vi "Handle Incoming Packets.vi"(8 "error in (no error)":errorcluster, 9 "SessionMailbox":refnum<queue>, 10 "Incoming Packet":refnum<class "ControlPacket.lvclass">, 11 "Server in":refnum<class "Server.lvclass">) -> (0 "error out":errorcluster, 1 "SessionMailbox out":refnum<queue>, 2 "Outgoing":T1, 3 "Server out":refnum<class "Server.lvclass">)   [LabVIEW 2013, in "MQTT Server.lvlib" / "Server.lvclass"]
uses:
  Server.lvclass
  <vilib>/LabVIEW Open Source Project/MQTT Control Packets/Control Packets/ControlPacket/ControlPacket.lvclass
  <vilib>/LabVIEW Open Source Project/MQTT Connection/MQTT_Base/Base Class/Response -- cluster.ctl
  <vilib>/LabVIEW Open Source Project/MQTT Connection/MQTT_Base/Base Class/MQTT_Base.lvclass
  <vilib>/LabVIEW Open Source Project/MQTT Control Packets/Control Packets/CONNECT/CONNECT.lvclass
  <vilib>/LabVIEW Open Source Project/MQTT Control Packets/Control Packets/CONNACK/Connect Return Code -- enum.ctl
  <vilib>/LabVIEW Open Source Project/MQTT Control Packets/Control Packets/DISCONNECT/DISCONNECT.lvclass
  <vilib>/LabVIEW Open Source Project/MQTT Control Packets/Control Packets/PUBLISH/PUBLISH.lvclass
  <vilib>/LabVIEW Open Source Project/MQTT Control Packets/Control Packets/PUBREL/PUBREL.lvclass
  <vilib>/LabVIEW Open Source Project/MQTT Control Packets/Control Packets/SUBSCRIBE/SUBSCRIBE.lvclass
  <vilib>/LabVIEW Open Source Project/MQTT Control Packets/Control Packets/ControlPacket/ControlPacket.lvclass/ControlPacket.ctl
  <vilib>/LabVIEW Open Source Project/MQTT Control Packets/Control Packets/SUBACK/Subscription Success Code.ctl
  <vilib>/LabVIEW Open Source Project/MQTT Control Packets/Control Packets/ControlPacket/QualityOfService -- enum.ctl
  <vilib>/LabVIEW Open Source Project/MQTT Control Packets/Control Packets/UNSUBSCRIBE/UNSUBSCRIBE.lvclass
  <vilib>/LabVIEW Open Source Project/MQTT Control Packets/Control Packets/PINGREQ/PINGREQ.lvclass
  <vilib>/LabVIEW Open Source Project/MQTT Control Packets/Control Packets/CONNACK/CONNACK.lvclass
  <vilib>/LabVIEW Open Source Project/MQTT Control Packets/Control Packets/SUBACK/SUBACK.lvclass
  <vilib>/LabVIEW Open Source Project/MQTT Control Packets/Control Packets/PINGRESP/PINGRESP.lvclass
  <vilib>/LabVIEW Open Source Project/MQTT Control Packets/Control Packets/UNSUBACK/UNSUBACK.lvclass
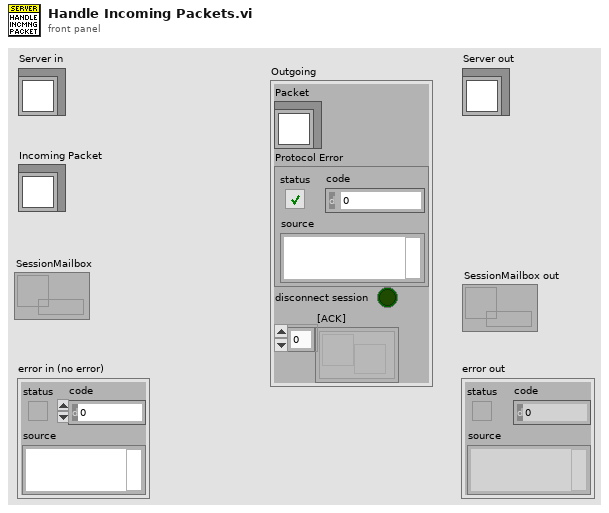
[diagram p1: front panel]
types:
  T1 = typedef "MQTT Base.lvlib/MQTT_Base.lvclass/Response -- cluster.ctl" = cluster{"Packet":refnum<class "ControlPacket.lvclass">, "Protocol Error":errorcluster, "disconnect session":bool, "[ACK]":refnum<notifier>[]}
  T2 = typedef "MQTT_Control_Packets.lvlib/CONNACK.lvclass/Connect Return Code -- enum.ctl" = enum16{"Connection accepted", "Unacceptable protocol version", "Identifier Rejected", "Server Unavailable", "Bad Username or Password", "Not Authorized"}
  T3 = typedef "MQTT_Control_Packets.lvlib/SUBACK.lvclass/Subscription Success Code.ctl" = cluster{"Subscription Failure":bool, "QoS":T4}
  T4 = typedef "MQTT_Control_Packets.lvlib/ControlPacket.lvclass/QualityOfService -- enum.ctl" = enum16{"0 (At Most Once)", "1 (At Least Once)", "2 (Exactly Once)"}
  T5 = typedef "MQTT_Control_Packets.lvlib/ControlPacket.lvclass/Control Packet Type -- enum.ctl" = enum16{"Reserved", "CONNECT", "CONNACK", "PUBLISH", "PUBACK", "PUBREC", "PUBREL", "PUBCOMP", "SUBSCRIBE", "SUBACK", "UNSUBSCRIBE", "UNSUBACK", "PINGREQ", "PINGRESP", "DISCONNECT", "AUTH"}
  T6 = typedef "MQTT_Control_Packets.lvlib/CONNECT.lvclass/ConnectFlags -- cluster.ctl" = cluster{"Reserved":bool, "Clean Session":bool, "Will Flag":bool, "Will QoS 1":bool, "Will QoS 2":bool, "Will Retain":bool, "Password Flag":bool, "User Name Flag":bool}
  T7 = typedef "MQTT_Control_Packets.lvlib/CONNECT.lvclass/ConnectPayload -- cluster.ctl" = cluster{"Will Topic":string, "Will Message":string, "Username":string, "Password":string}
  T8 = typedef "MQTT_Control_Packets.lvlib/SUBSCRIBE.lvclass/Topic Subscription -- cluster.ctl" = cluster{"Topic Filter":string, "QoS":T4}
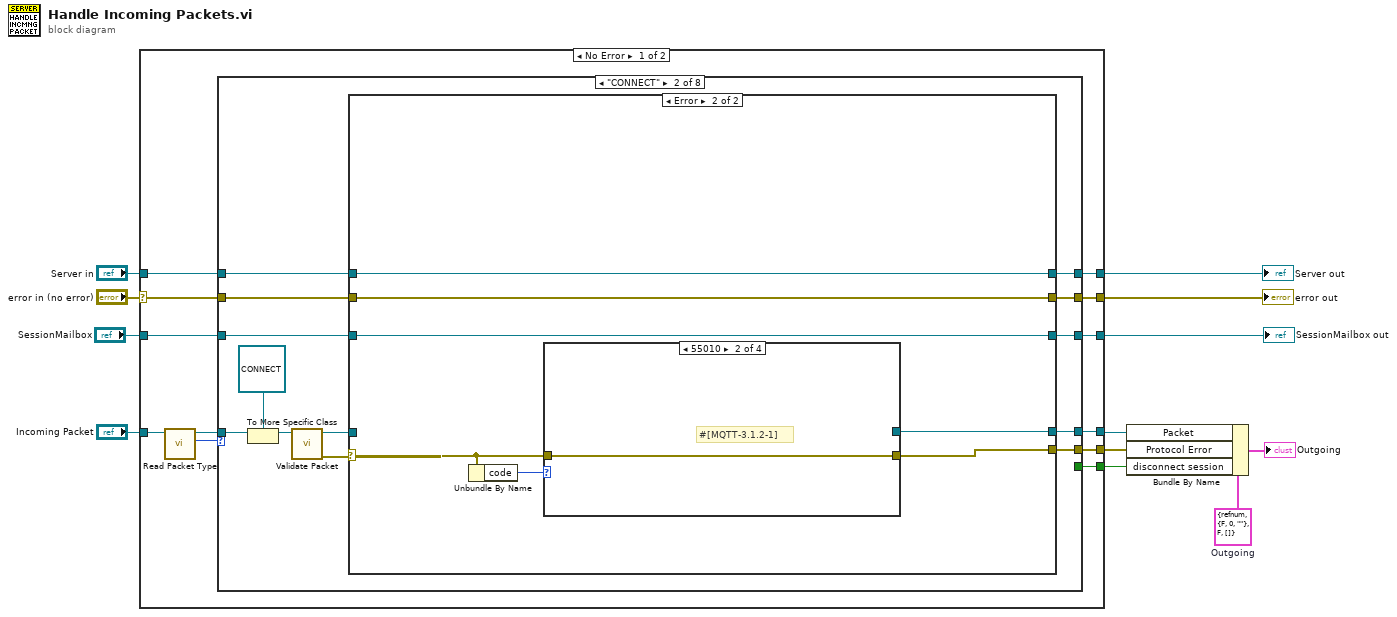
[diagram p0: block diagram]
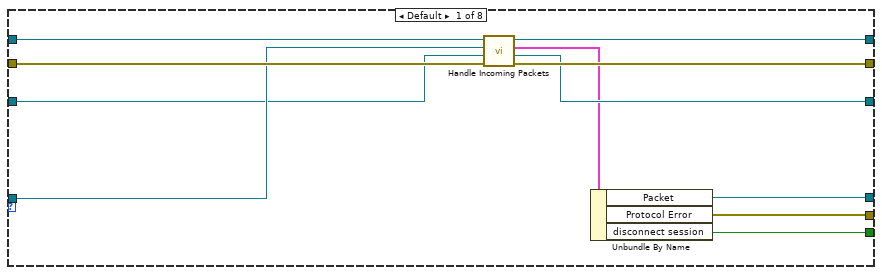
[diagram p2: hidden frame]
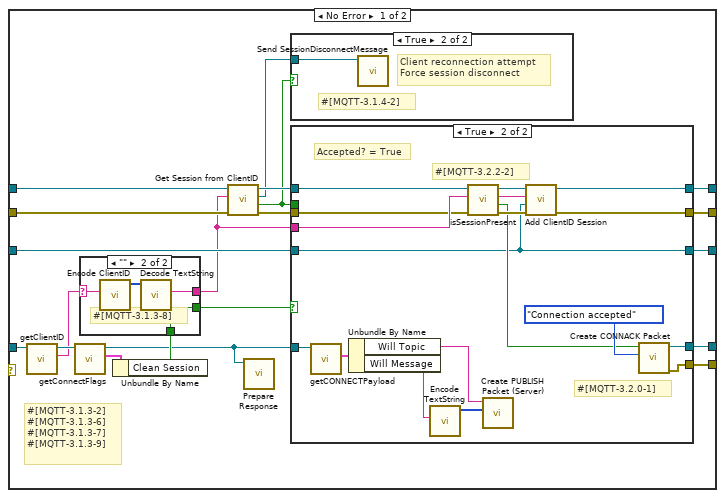
[diagram p3: hidden frame]
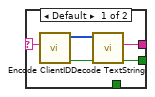
[diagram p4: hidden frame]
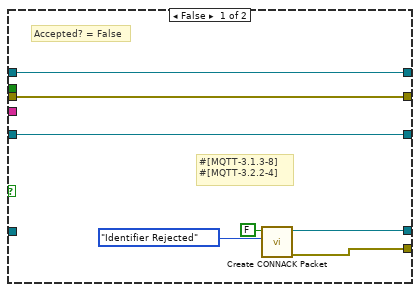
[diagram p6: hidden frame]
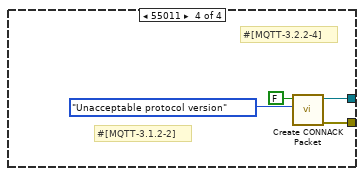
[diagram p9: hidden frame]
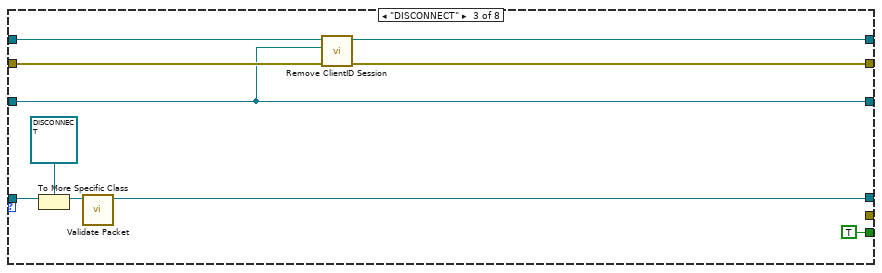
[diagram p10: hidden frame]
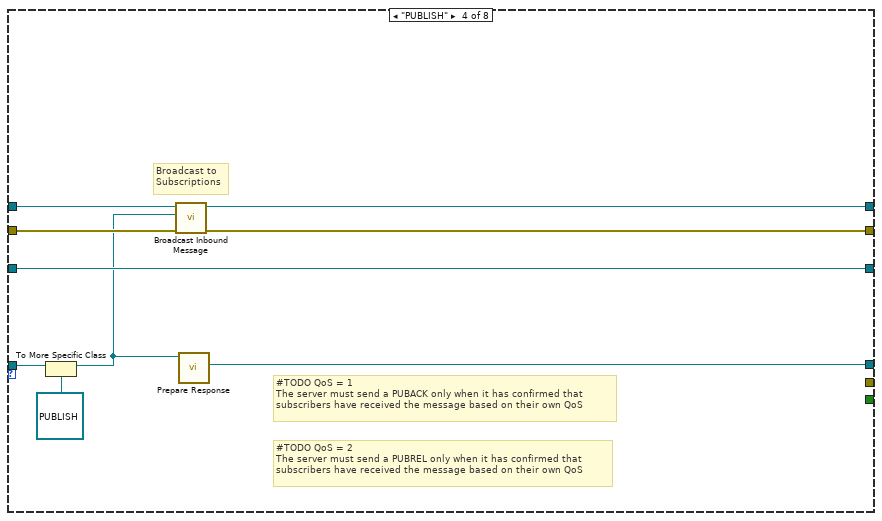
[diagram p11: hidden frame]
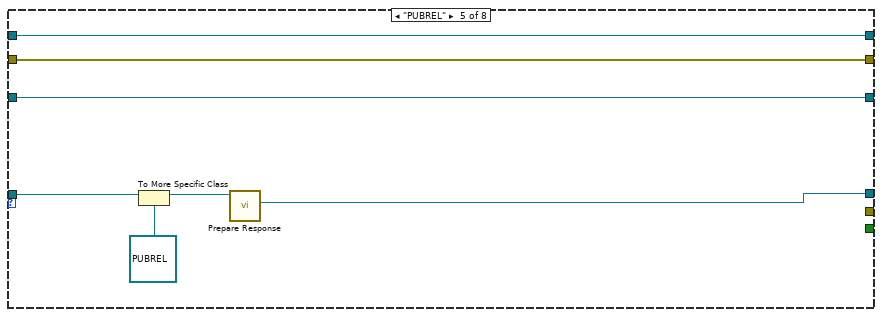
[diagram p12: hidden frame]
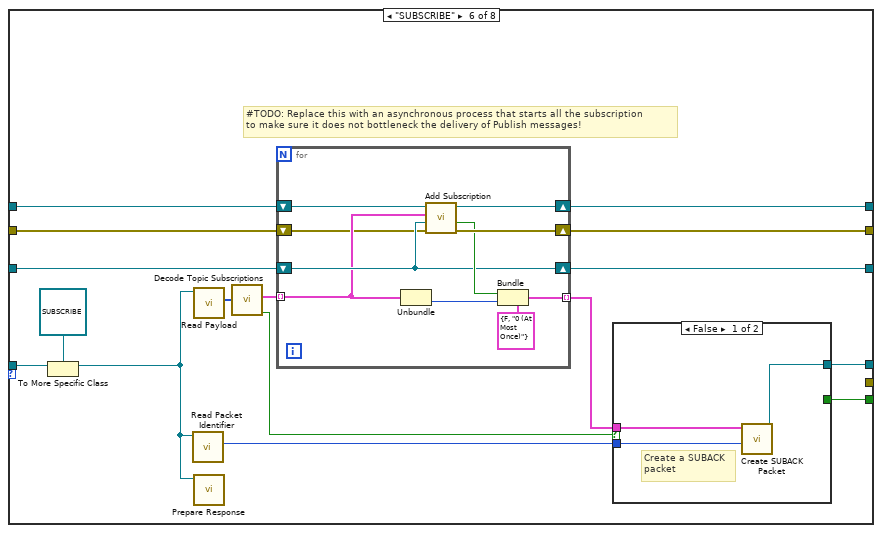
[diagram p13: hidden frame]
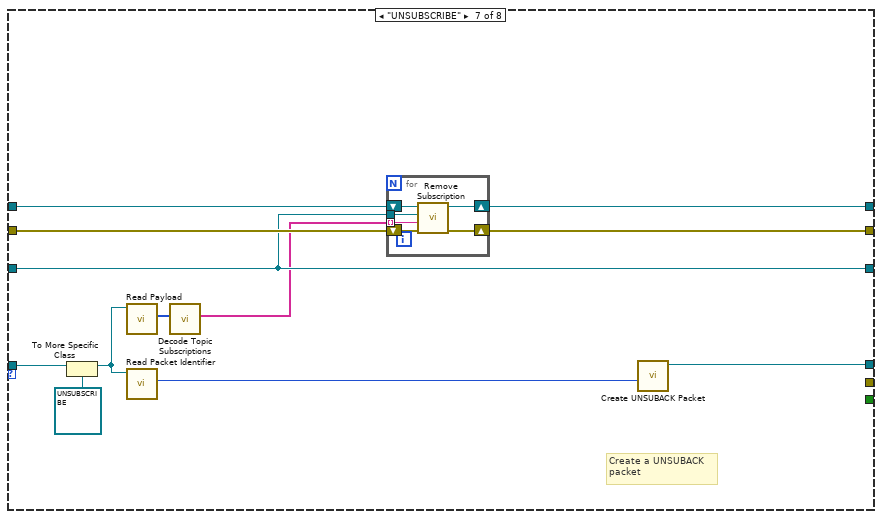
[diagram p15: hidden frame]
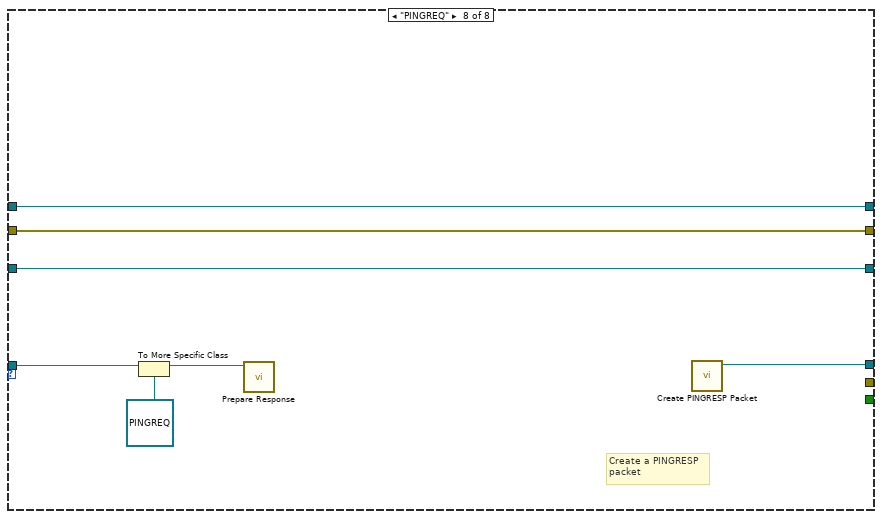
[diagram p16: hidden frame]
diagram:
  w7 = T1 {"Packet"=refnum, "Protocol Error"={"status"=FALSE, "code"=0, "source"=""}, "disconnect session"=FALSE, "[ACK]"=[]}  # Outgoing
  n1 = case shown="No Error" "error in (no error)" {
    selector: "error in (no error)" -> [w22 w200]
    tunnel: [w19 w200] -> w11
    tunnel: [w20 w199] -> w9
    tunnel: "Server in" -> [w21 w199]
    tunnel: "Incoming Packet" -> [w15 _]
    tunnel: [w18 _] -> w6
    tunnel: [w17 _] -> w2
    tunnel: "SessionMailbox" -> [w16 w198]
    tunnel: [w14 w198] -> w1
    tunnel: [w13 _] -> w4
    frame No Error {
      n2 = call <vilib>:"Read Packet Type.vi"("ControlPacket in"=w15) -> ("Control Packet Type"=w24:T5, "ControlPacket out"=w23:refnum<class "ControlPacket.lvclass">)  [unwired: 9 in]
      n3 = case shown="\"CONNECT\"" w24 {
        tunnel: w23 -> [w31 w45 w126 w134 w139 w158 w184 w194]
        tunnel: w22 -> [w33 w42 w121 w132 w141 w148 w180 w196]
        tunnel: w21 -> [w35 w43 w123 w130 w142 w151 w178 w197]
        tunnel: [w34 w40 w122 w129 w142 w150 w177 w197] -> w20
        tunnel: [w32 w41 w120 w131 w141 w149 w179 w196] -> w19
        tunnel: w16 -> [w30 w39 w119 w135 w140 w147 w176 w195]
        tunnel: [w27 w38 w117 w127 w136 w152 w174 w193] -> w18
        tunnel: [w26 w37 _ _ _ _ _ _] -> w17
        tunnel: [w29 w36 w119 w135 w140 w146 w176 w195] -> w14
        tunnel: [w25 _ TRUE ("disconnect session") _ _ w144 _ _] -> w13
        frame Default {
          n4 = call-parent "Handle Incoming Packets.vi"("error in (no error)"=w33, "SessionMailbox"=w30, "Incoming Packet"=w31, "MQTT_Base in"=w35) -> ("error out"=w32:errorcluster, "SessionMailbox out"=w29:refnum<queue>, "Outgoing"=w28:T1, "MQTT_Base out"=w34:refnum<class "Server.lvclass">)  [unwired: 4 in]
          n5 = Unbundle By Name(w28) -> ("Packet"=w27:refnum<class "ControlPacket.lvclass">, "Protocol Error"=w26:errorcluster, "disconnect session"=w25:bool)
        }
        frame "CONNECT" {
          n6 = To More Specific Class(target class=refnum<class "CONNECT.lvclass"> refnum ("CONNECT.lvclass"), reference=w45) -> (specific class reference=w44:refnum<class "CONNECT.lvclass">)  [unwired: 1 in, 1 out]
          n7 = call <vilib>:"Validate Packet.vi"("ControlPacket in"=w44) -> ("error out"=w48:errorcluster, "ControlPacket out"=w47:refnum<class "CONNECT.lvclass">)  [unwired: 9 in]
          n8 = case shown="Error" w48 {
            selector: w48 -> [_ w108]
            tunnel: w47 -> [w68 _]
            tunnel: w43 -> [w64 w107]
            tunnel: w42 -> [w62 w106]
            tunnel: [w66 w106] -> w41
            tunnel: [w67 w107] -> w40
            tunnel: w39 -> [w65 w103]
            tunnel: [w59 w105] -> w38
            tunnel: [w58 w104] -> w37
            tunnel: [w56 w103] -> w36
            frame No Error {
              # "#[MQTT-3.1.3-2]\n#[MQTT-3.1.3-6]\n#[MQTT-3.1.3-7]\n#[MQTT-3.1.3-9]"
              n9 = call <vilib>:"getClientID.vi"("CONNECT in"=w68) -> ("Client ID"=w51:string, "CONNECT out"=w55:refnum<class "CONNECT.lvclass">)  [unwired: 9 in]
              n10 = call <vilib>:"getConnectFlags.vi"("CONNECT in"=w55) -> ("Connect Flags"=w54:T6, "CONNECT out"=w49:refnum<class "CONNECT.lvclass">)  [unwired: 9 in]
              n11 = Unbundle By Name(w54) -> ("Clean Session"=w52:bool)
              n12 = case shown="\"\"" w51 {
                selector: w51 -> [w72 w75]
                tunnel: [w71 w76] -> w53
                tunnel: w52 -> [_ w76]
                tunnel: [w69 w73] -> w50
                frame Default {
                  n13 = call <vilib>:"Encode ClientID.vi"("Client ID (empty: generate new)"=w72) -> ("valid Client ID"=w71:bool, "Length-Prefixed Field"=w70:u8[])  [unwired: 9 in]
                  n14 = call <vilib>:"Decode TextString.vi"("Length-Prefixed Field"=w70) -> ("Text String"=w69:string)  [unwired: 8 in, 2 out]
                }
                frame "" {
                  # "#[MQTT-3.1.3-8]"
                  n15 = call <vilib>:"Encode ClientID.vi"("Client ID (empty: generate new)"=w75) -> ("Length-Prefixed Field"=w74:u8[])  [unwired: 9 in, 1 out]
                  n16 = call <vilib>:"Decode TextString.vi"("Length-Prefixed Field"=w74) -> ("Text String"=w73:string)  [unwired: 8 in, 2 out]
                }
              }
              n17 = call "Get Session from ClientID.vi"("error in (no error)"=w62, "Client ID"=w50, "MQTT Server"=w64) -> ("error out"=w61:errorcluster, "found?"=w57:bool, "SessionMailbox"=w60:refnum<queue>, "MQTT Server"=w63:refnum<class "Server.lvclass">)  [unwired: 5 in]
              n18 = call-dynamic "Prepare Response.vi"("ControlPacket in"=w49) -> ()  [unwired: 7 in, 4 out]
              n19 = case shown="True" w57 {
                tunnel: w60 -> [_ w77]
                frame False {
                }
                frame True {
                  # "#[MQTT-3.1.4-2]"
                  # "Client reconnection attempt\nForce session disconnect"
                  n20 = call "Send SessionDisconnectMessage.vi"("SessionMailbox"=w77) -> ()  [unwired: 10 in, 1 out]
                }
              }
              n21 = case shown="True" w53 {
                tunnel: [w82 w101] -> w67
                tunnel: [w81 w100] -> w66
                tunnel: w65 -> [w78 w90]
                tunnel: w63 -> [w82 w92]
                tunnel: w61 -> [w81 w91]
                tunnel: w50 -> [_ w96]
                tunnel: [w80 w99] -> w59
                tunnel: [w79 w98] -> w58
                tunnel: w57 -> [_ _]
                tunnel: [w78 w90] -> w56
                tunnel: w49 -> [_ w89]
                frame False {
                  # "Accepted? = False"
                  # "#[MQTT-3.1.3-8]\n#[MQTT-3.2.2-4]"
                  n22 = call <vilib>:"Create CONNACK Packet.vi"("Return Code"=Connect_Return_Code_--_enum."Identifier Rejected", "Session Present"=FALSE) -> ("error out"=w79:errorcluster, "CONNACK"=w80:refnum<class "CONNACK.lvclass">)  [unwired: 7 in, 1 out]
                }
                frame True {
                  # "Accepted? = True"
                  # "#[MQTT-3.2.2-2]"
                  # "#[MQTT-3.2.0-1]"
                  n23 = call <vilib>:"getCONNECTPayload.vi"("CONNECT in"=w89) -> ("Payload"=w88:T7)  [unwired: 9 in, 1 out]
                  n24 = Unbundle By Name(w88) -> ("Will Topic"=w87:string, "Will Message"=w85:string)
                  n25 = call <vilib>:"Encode TextString.vi"("Text String"=w85) -> ("Length-Prefixed Field"=w86:u8[])  [unwired: 10 in]
                  n26 = call "isSessionPresent.vi"("error in"=w91, "Client ID"=w96, "MQTT Server"=w92) -> ("error out"=w97:errorcluster, "Session Present"=w94:bool, "Client ID dup"=w95:string, "MQTT Server out"=w93:refnum<class "Server.lvclass">)  [unwired: 5 in]
                  n27 = call <vilib>:"Create PUBLISH Packet (Server).vi"("Payload"=w86, "Topic Name"=w87) -> ()  [unwired: 6 in, 4 out]
                  n28 = call "Add ClientID Session.vi"("error in (no error)"=w97, "SessionMailbox"=w90, "Client ID"=w95, "MQTT Server"=w93) -> ("error out"=w100:errorcluster, "MQTT Server"=w101:refnum<class "Server.lvclass">)  [unwired: 6 in]
                  n29 = call <vilib>:"Create CONNACK Packet.vi"("Return Code"=Connect_Return_Code_--_enum."Connection accepted", "Session Present"=w94) -> ("error out"=w98:errorcluster, "CONNACK"=w99:refnum<class "CONNACK.lvclass">)  [unwired: 7 in, 1 out]
                }
              }
            }
            frame Error {
              n30 = Unbundle By Name(w108) -> ("code"=w109:i32)
              n31 = case shown="55010" w109 {
                tunnel: [_ _ _ w114] -> w105
                tunnel: [w110 w111 w112 w113] -> w104
                tunnel: w108 -> [w110 w111 w112 _]
                frame Default {
                  # "#[MQTT-3.1.4-1]"
                  # "Any unhandled error should be\nthralled to the Protocol error terminal"
                }
                frame 55010 {
                  # "#[MQTT-3.1.2-1]"
                }
                frame 55012 {
                  # "#[MQTT-3.1.2-3]"
                }
                frame 55011 {
                  # "#[MQTT-3.2.2-4]"
                  # "#[MQTT-3.1.2-2]"
                  n32 = call <vilib>:"Create CONNACK Packet.vi"("Return Code"=Connect_Return_Code_--_enum."Unacceptable protocol version", "Session Present"=FALSE) -> ("error out"=w113:errorcluster, "CONNACK"=w114:refnum<class "CONNACK.lvclass">)  [unwired: 7 in, 1 out]
                }
              }
            }
          }
        }
        frame "DISCONNECT" {
          n33 = To More Specific Class(target class=refnum<class "DISCONNECT.lvclass"> refnum ("DISCONNECT.lvclass"), reference=w126) -> (specific class reference=w125:refnum<class "DISCONNECT.lvclass">)  [unwired: 1 in, 1 out]
          n34 = call <vilib>:"Validate Packet.vi"("ControlPacket in"=w125) -> ("ControlPacket out"=w117:refnum<class "DISCONNECT.lvclass">)  [unwired: 9 in, 1 out]
          n35 = call "Remove ClientID Session.vi"("error in (no error)"=w121, "SessionMailbox"=w119, "MQTT Server"=w123) -> ("error out"=w120:errorcluster, "MQTT Server"=w122:refnum<class "Server.lvclass">)  [unwired: 7 in]
        }
        frame "PUBLISH" {
          # "#TODO QoS = 1\nThe server must send a PUBACK only when it has confirmed that\nsubscribers have received the message based on their own QoS"
          # "#TODO QoS = 2\nThe server must send a PUBREL only when it has confirmed that\nsubscribers have received the message based on their own QoS"
          # "Broadcast to\nSubscriptions"
          n36 = To More Specific Class(target class=refnum<class "PUBLISH.lvclass"> refnum ("PUBLISH.lvclass"), reference=w134) -> (specific class reference=w128:refnum<class "PUBLISH.lvclass">)  [unwired: 1 in, 1 out]
          n37 = call <vilib>:"Broadcast Inbound Message.vi"("error in (no error)"=w132, "Inbound Message"=w128, "MQTT_Base in"=w130) -> ("error out"=w131:errorcluster, "MQTT_Base out"=w129:refnum<class "Server.lvclass">)  [unwired: 7 in]
          n38 = call-dynamic "Prepare Response.vi"("PUBLISH in"=w128) -> ("ControlPacket response"=w127:refnum<class "ControlPacket.lvclass">)  [unwired: 7 in, 3 out]
        }
        frame "PUBREL" {
          n39 = To More Specific Class(target class=refnum<class "PUBREL.lvclass"> refnum ("PUBREL.lvclass"), reference=w139) -> (specific class reference=w137:refnum<class "PUBREL.lvclass">)  [unwired: 1 in, 1 out]
          n40 = call-dynamic "Prepare Response.vi"("PUBREL in"=w137) -> ("ControlPacket response"=w136:refnum<class "ControlPacket.lvclass">)  [unwired: 7 in, 3 out]
        }
        frame "SUBSCRIBE" {
          # "#TODO: Replace this with an asynchronous process that starts all the subscription\nto make sure it does not bottleneck the delivery of Publish messages!"
          n41 = To More Specific Class(target class=refnum<class "SUBSCRIBE.lvclass"> refnum ("SUBSCRIBE.lvclass"), reference=w158) -> (specific class reference=w143:refnum<class "SUBSCRIBE.lvclass">)  [unwired: 1 in, 1 out]
          n42 = call <vilib>:"Read Packet Identifier.vi"("ControlPacket in"=w143) -> ("Packet Identifier"=w155:u16)  [unwired: 9 in, 1 out]
          n43 = call <vilib>:"Read Payload.vi"("ControlPacket in"=w143) -> ("Payload"=w156:u8[])  [unwired: 9 in, 1 out]
          n44 = call-dynamic "Prepare Response.vi"("ControlPacket in"=w143) -> ()  [unwired: 7 in, 4 out]
          n45 = call <vilib>:"Decode Topic Subscriptions.vi"("Payload"=w156) -> ("invalid UTF8"=w145:bool, "Topic Subscriptions"=w154:T8[])  [unwired: 8 in, 1 out]
          n46 = for {
            tunnel: w154 -> [w165] mode=indexing
            tunnel: [w172] -> w153 mode=indexing
            shift-right: [w168] -> w150
            shift-left: w151 -> [w164]
            shift-right: [w169] -> w149
            shift-left: w148 -> [w163]
            shift-right: [w166] -> w146
            shift-left: w147 -> [w166]
            n47 = Unbundle(w165) -> ("QoS"=w170:T4)  [unwired: 1 out]
            n48 = call <vilib>:"Add Subscription.vi"("error in (no error)"=w163, "SessionMailbox"=w166, "Topic Subscription"=w165, "MQTT_Base in"=w164) -> ("error out"=w169:errorcluster, "Failed"=w167:bool, "MQTT_Base out"=w168:refnum<class "Server.lvclass">)  [unwired: 5 in]
            n49 = Bundle(cluster=T3 {"Subscription Failure"=FALSE, "QoS"=enum."0 (At Most Once)"} ("Topic Subscription"), "Subscription Failure"=w167, "QoS"=w170) -> (w172:T3)
          }
          n50 = case shown="False" w145 {
            selector: w145 -> [_ w162]
            tunnel: w155 -> [w161 _]
            tunnel: w153 -> [w160 _]
            tunnel: [w159 _] -> w152
            tunnel: [_ w162] -> w144
            frame False {
              # "Create a SUBACK\npacket"
              n51 = call <vilib>:"Create SUBACK Packet.vi"("Packet ID"=w161, "Return Codes"=w160) -> ("SUBACK"=w159:refnum<class "SUBACK.lvclass">)  [unwired: 7 in, 2 out]
            }
            frame True {
              # "Invalid UTF8 string"
            }
          }
        }
        frame "UNSUBSCRIBE" {
          # "Create a UNSUBACK\npacket"
          n52 = To More Specific Class(target class=refnum<class "UNSUBSCRIBE.lvclass"> refnum ("UNSUBSCRIBE.lvclass"), reference=w184) -> (specific class reference=w183:refnum<class "UNSUBSCRIBE.lvclass">)  [unwired: 1 in, 1 out]
          n53 = call <vilib>:"Read Payload.vi"("ControlPacket in"=w183) -> ("Payload"=w181:u8[])  [unwired: 9 in, 1 out]
          n54 = call <vilib>:"Read Packet Identifier.vi"("ControlPacket in"=w183) -> ("Packet Identifier"=w173:u16)  [unwired: 9 in, 1 out]
          n55 = call <vilib>:"Decode Topic Subscriptions.vi"("Payload"=w181) -> ("Topic Subscriptions"=w175:string[])  [unwired: 9 in, 1 out]
          n56 = for {
            tunnel: w176 -> [w186]
            shift-right: [w187] -> w177
            shift-left: w178 -> [w188]
            shift-right: [w189] -> w179
            shift-left: w180 -> [w190]
            tunnel: w175 -> [w185] mode=indexing
            n57 = call <vilib>:"Remove Subscription.vi"("error in (no error)"=w190, "Topic Filter"=w185, "SessionMailbox"=w186, "MQTT_Base in"=w188) -> ("error out"=w189:errorcluster, "MQTT_Base out"=w187:refnum<class "Server.lvclass">)  [unwired: 5 in, 1 out]
          }
          n58 = call <vilib>:"Create UNSUBACK Packet.vi"("Packet ID"=w173) -> ("UNSUBACK out"=w174:refnum<class "UNSUBACK.lvclass">)  [unwired: 8 in, 2 out]
        }
        frame "PINGREQ" {
          # "Create a PINGRESP\npacket"
          n59 = To More Specific Class(target class=refnum<class "PINGREQ.lvclass"> refnum ("PINGREC.lvclass"), reference=w194) -> (specific class reference=w191:refnum<class "PINGREQ.lvclass">)  [unwired: 1 in, 1 out]
          n60 = call-dynamic "Prepare Response.vi"("PINGREQ in"=w191) -> ()  [unwired: 7 in, 4 out]
          n61 = call <vilib>:"Create PINGRESP Packet.vi"() -> ("PINGRESP out"=w193:refnum<class "PINGRESP.lvclass">)  [unwired: 9 in, 2 out]
        }
      }
    }
    frame Error {
    }
  }
  "error out" <- w11
  "Server out" <- w9
  "SessionMailbox out" <- w1
  n62 = Bundle By Name(cluster=w7, "Packet"=w6, "Protocol Error"=w2, "disconnect session"=w4) -> (→"Outgoing":T1)
